vi "set Additional ResponseEvent.vi"(0 "LVx in":refnum<class "LVx.lvclass">, 5 "Fire Additional Event for Response?":bool=TRUE, 11 "error in (no error)":errorcluster) -> (4 "LVx out":refnum<class "LVx.lvclass">, 15 "error out":errorcluster)   [LabVIEW 2011, in "LVx.lvlib" / "LVx.lvclass"]
uses:
  LVx.lvclass
  LVx.lvclass/LVx.ctl
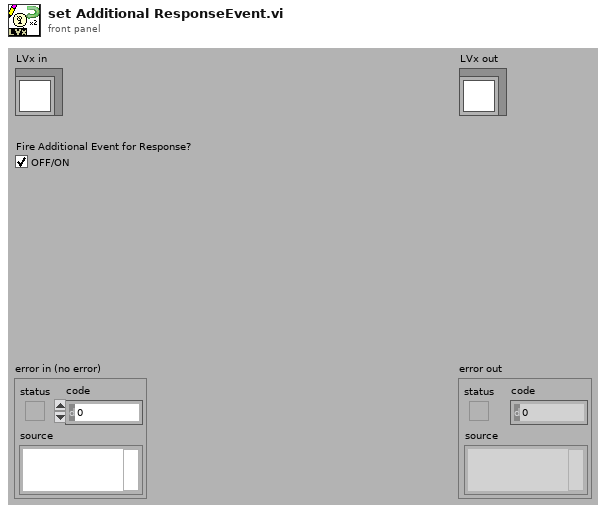
[diagram p1: front panel]
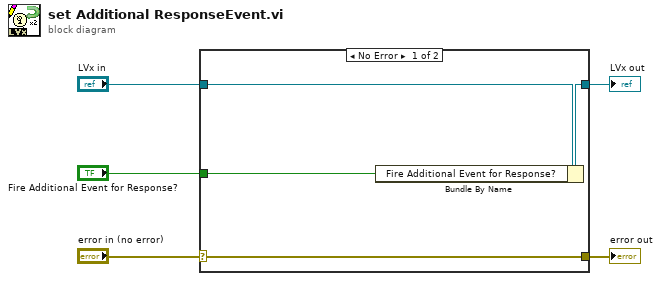
[diagram p0: block diagram]
diagram:
  n1 = case shown="No Error" "error in (no error)" {
    selector: "error in (no error)" -> [w9 w10]
    tunnel: [w9 w10] -> w4
    tunnel: [w7 w11] -> w2
    tunnel: "LVx in" -> [w8 w11]
    tunnel: "Fire Additional Event for Response?" -> [w6 _]
    frame No Error {
      n2 = Bundle By Name(cluster=w8, "Fire Additional Event for Response?"=w6) -> (w7:refnum<class "LVx.lvclass">)
    }
    frame Error {
    }
  }
  "error out" <- w4
  "LVx out" <- w2
